vi "Write RFSG Session.vi"(8 "error in (no error)":errorcluster, 10 "RFSG Session":refnum<k15>, 11 "Scalar Path in":refnum<class "Scalar Path.lvclass">) -> (0 "error out":errorcluster, 3 "Scalar Path out":refnum<class "Scalar Path.lvclass">)   [LabVIEW 2023, in "RFFixtureCharact.Public.lvlib" / "Scalar Path.lvclass"]
uses:
  Scalar Path.lvclass
  Scalar Path.lvclass/Scalar Path.ctl
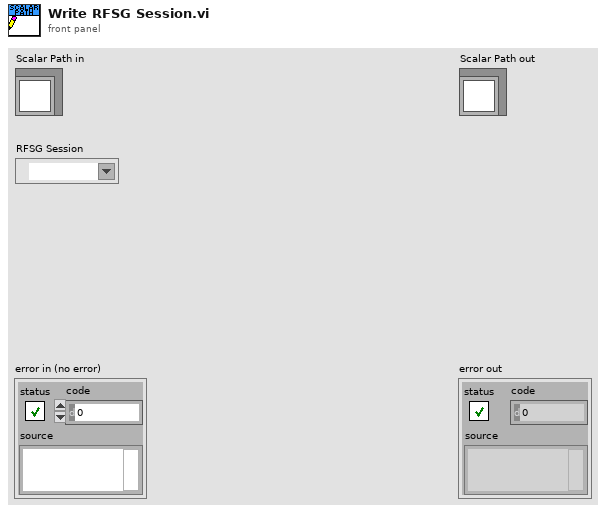
[diagram p1: front panel]
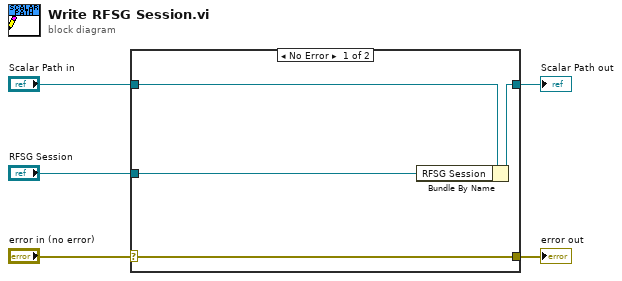
[diagram p0: block diagram]
diagram:
  n1 = case shown="No Error" "error in (no error)" {
    selector: "error in (no error)" -> [w9 w10]
    tunnel: [w9 w10] -> w4
    tunnel: [w7 w11] -> w2
    tunnel: "Scalar Path in" -> [w8 w11]
    tunnel: "RFSG Session" -> [w6 _]
    frame No Error {
      n2 = Bundle By Name(cluster=w8, "RFSG Session"=w6) -> (w7:refnum<class "Scalar Path.lvclass">)
    }
    frame Error {
    }
  }
  "error out" <- w4
  "Scalar Path out" <- w2
